vi "Write Zero Readings Strings.vi"(8 "error in (no error)":errorcluster, 11 "Zero Readings":cluster{"mean":dbl, "standard deviation":dbl}[](array[cluster])) -> (0 "error out":errorcluster, 3 "Results":T1[](array[typedef]))   [LabVIEW 2015]
uses:
  Controls/Test Info.ctl
panel:
  # "Filter Phase Average Std SamNum"
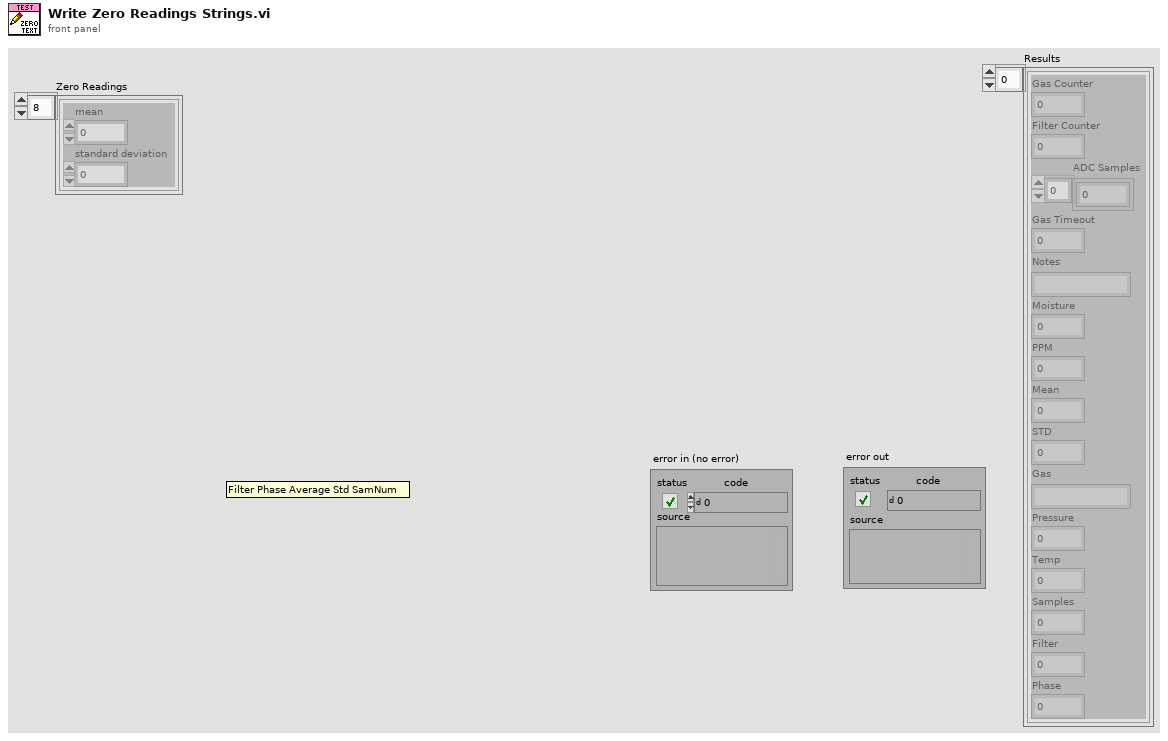
[diagram p1: front panel]
types:
  T1 = typedef "Test Info.ctl" = cluster{"Gas Counter":u16, "Filter Counter":u16, "ADC Samples":dbl[], "Gas Timeout":u16, "Notes":string, "Moisture":dbl, "PPM":dbl, "Mean":dbl, "STD":dbl, "Gas":string, "Pressure":dbl, "Temp":dbl, "Samples":u16, "Filter":u8, "Phase":dbl}
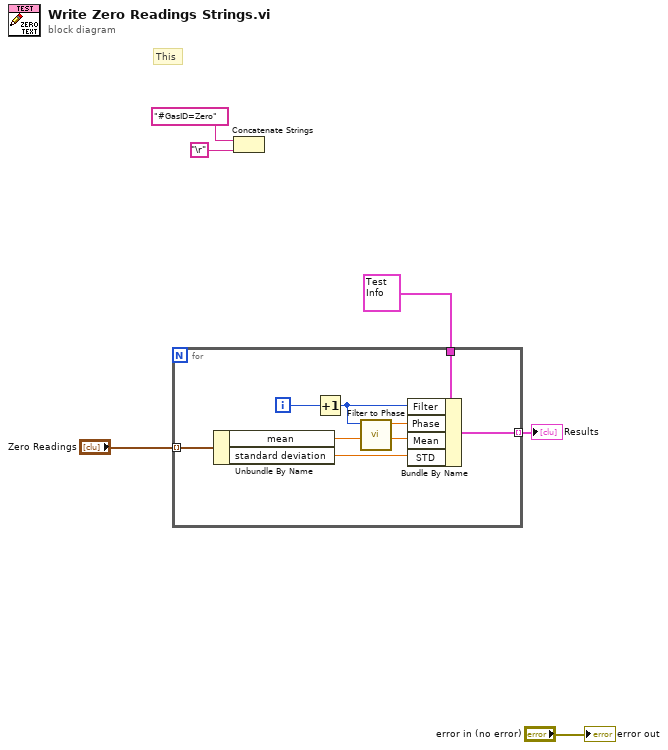
[diagram p0: block diagram]
diagram:
  # "This"
  n1 = for {
    tunnel: "Zero Readings" -> [w14] mode=indexing
    tunnel: T1 {"Gas Counter"=0, "Filter Counter"=0, "ADC Samples"=[], "Gas Timeout"=0, "Notes"="", "Moisture"=0.0, "PPM"=0.0, "Mean"=0.0, "STD"=0.0, "Gas"="", "Pressure"=0.0, "Temp"=0.0, "Samples"=0, "Filter"=0, "Phase"=0.0} ("Result") -> [w8]
    tunnel: [w7] -> w3 mode=indexing
    i -> [w13]
    n2 = Unbundle By Name(w14) -> ("mean"=w10:dbl, "standard deviation"=w9:dbl)
    n3 = Increment(x=w13) -> (x+1=w11:i32)
    n4 = call "Filter to Phase.vi"("Filter"=w11) -> ("Phase"=w12:dbl)  [unwired: 10 in]
    n5 = Bundle By Name(cluster=w8, "Filter"=w11, "Phase"=w12, "Mean"=w10, "STD"=w9) -> (w7:T1)
  }
  "Results" <- w3
  n6 = Concatenate Strings("#GasID=Zero", "\r") -> ()  [unwired: 1 out]
  "error out" <- "error in (no error)"
